vi "NyquistTrimCoefficients.vi"(7 "Cutoff type":string(combo), 9 "InterpolatedCoefficients":dbl[](array[numeric])=[1.0, 0.9893, 1.019, 1.0269, 1.0344, 1.0416, 1.0487, 1.0558, 1.0628, 1.0701, 1.0776, 1.0854, 1.0937, 1.1026, 1.1121, 1.1224, 1.1336, 1.1457, 1.1589, 1.1733, 1.189, 1.2061, 1.2246, 1.2447, 1.2662, 1.289, 1.3129, 1.3376, 1.3632, 1.3892, 1.4157, 1.4425, 1.4693, 1.496, 1.5226, 1.5491, 1.5754, 1.6016, 1.6277, 1.6535, 1.6792, 1.7046, 1.7298, 1.7548, 1.7794, 1.8033, 1.8263, 1.8483, 1.869, 1.8882, 1.9058, 1.9215, 1.935, 1.9464, 1.9556, 1.9628, 1.9684, 1.9723, 1.9748, 1.9762, 1.9765, 1.9759, 1.9748, 1.9731, 1.9711, 1.9689, 1.9667, 1.9646, 1.9628, 1.9614, 1.9606, 1.9605, 1.9612, 1.963, 1.9657, 1.9693, 1.9738, 1.979, 1.9848, 1.9913, 1.9983, 2.0059, 2.0138, 2.0221, 2.0308, 2.0401, 2.05, 2.0607, 2.0722, 2.0847, 2.0983, 2.113, 0.0, 0.0, 0.0, 0.0, 0.0, 0.0, 0.0, 0.0, 0.0, 0.0, 0.0, 0.0, 0.0, 0.0, 0.0, 0.0, 0.0, 0.0, 0.0, 0.0, 0.0, 0.0, 0.0, 0.0, 0.0, 0.0, 0.0, 0.0, 0.0, 0.0, 0.0, 0.0, 0.0, 0.0, 0.0, 0.0, 0.0, 0.0, 0.0, 0.0, 0.0, 0.0, 0.0, 0.0, 0.0, 0.0, 0.0, 0.0, 0.0, 0.0, 0.0, 0.0], 10 "Frequencies":dbl[](array[numeric])=[1.0, 0.9893, 1.019, 1.0269, 1.0344, 1.0416, 1.0487, 1.0558, 1.0628, 1.0701, 1.0776, 1.0854, 1.0937, 1.1026, 1.1121, 1.1224, 1.1336, 1.1457, 1.1589, 1.1733, 1.189, 1.2061, 1.2246, 1.2447, 1.2662, 1.289, 1.3129, 1.3376, 1.3632, 1.3892, 1.4157, 1.4425, 1.4693, 1.496, 1.5226, 1.5491, 1.5754, 1.6016, 1.6277, 1.6535, 1.6792, 1.7046, 1.7298, 1.7548, 1.7794, 1.8033, 1.8263, 1.8483, 1.869, 1.8882, 1.9058, 1.9215, 1.935, 1.9464, 1.9556, 1.9628, 1.9684, 1.9723, 1.9748, 1.9762, 1.9765, 1.9759, 1.9748, 1.9731, 1.9711, 1.9689, 1.9667, 1.9646, 1.9628, 1.9614, 1.9606, 1.9605, 1.9612, 1.963, 1.9657, 1.9693, 1.9738, 1.979, 1.9848, 1.9913, 1.9983, 2.0059, 2.0138, 2.0221, 2.0308, 2.0401, 2.05, 2.0607, 2.0722, 2.0847, 2.0983, 2.113, 0.0, 0.0, 0.0, 0.0, 0.0, 0.0, 0.0, 0.0, 0.0, 0.0, 0.0, 0.0, 0.0, 0.0, 0.0, 0.0, 0.0, 0.0, 0.0, 0.0, 0.0, 0.0, 0.0, 0.0, 0.0, 0.0, 0.0, 0.0, 0.0, 0.0, 0.0, 0.0, 0.0, 0.0, 0.0, 0.0, 0.0, 0.0, 0.0, 0.0, 0.0, 0.0, 0.0, 0.0, 0.0, 0.0, 0.0, 0.0, 0.0, 0.0, 0.0, 0.0], 11 "fs (Hz)":dbl) -> (1 "NyquistLimitedCoefficients":dbl[](array[numeric])=[1.0, 0.9893, 1.019, 1.0269, 1.0344, 1.0416, 1.0487, 1.0558, 1.0628, 1.0701, 1.0776, 1.0854, 1.0937, 1.1026, 1.1121, 1.1224, 1.1336, 1.1457, 1.1589, 1.1733, 1.189, 1.2061, 1.2246, 1.2447, 1.2662, 1.289, 1.3129, 1.3376, 1.3632, 1.3892, 1.4157, 1.4425, 1.4693, 1.496, 1.5226, 1.5491, 1.5754, 1.6016, 1.6277, 1.6535, 1.6792, 1.7046, 1.7298, 1.7548, 1.7794, 1.8033, 1.8263, 1.8483, 1.869, 1.8882, 1.9058, 1.9215, 1.935, 1.9464, 1.9556, 1.9628, 1.9684, 1.9723, 1.9748, 1.9762, 1.9765, 1.9759, 1.9748, 1.9731, 1.9711, 1.9689, 1.9667, 1.9646, 1.9628, 1.9614, 1.9606, 1.9605, 1.9612, 1.963, 1.9657, 1.9693, 1.9738, 1.979, 1.9848, 1.9913, 1.9983, 2.0059, 2.0138, 2.0221, 2.0308, 2.0401, 2.05, 2.0607, 2.0722, 2.0847, 2.0983, 2.113, 0.0, 0.0, 0.0, 0.0, 0.0, 0.0, 0.0, 0.0, 0.0, 0.0, 0.0, 0.0, 0.0, 0.0, 0.0, 0.0, 0.0, 0.0, 0.0, 0.0, 0.0, 0.0, 0.0, 0.0, 0.0, 0.0, 0.0, 0.0, 0.0, 0.0, 0.0, 0.0, 0.0, 0.0, 0.0, 0.0, 0.0, 0.0, 0.0, 0.0, 0.0, 0.0, 0.0, 0.0, 0.0, 0.0, 0.0, 0.0, 0.0, 0.0, 0.0, 0.0], 3 "NyquistFreq":dbl)   [LabVIEW 2011]
uses:
  <vilib>/Analysis/NI_AALBase.lvlib
panel:
  in  "cosineFadeLength":i32=12
  out "XY Graph":cluster{"Frequencies":dbl[], dbl[]}[](graph)
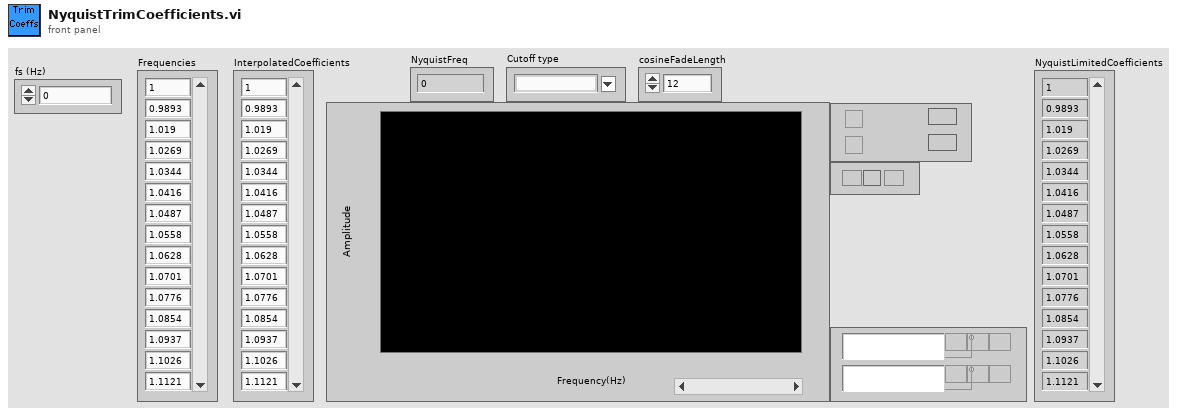
[diagram p1: front panel]
types:
  T1 = cluster{"Frequencies":dbl[], "InterpolatedCoefficients":dbl[]}
  T2 = cluster{"Frequencies":dbl[], "InterpolatedCoefficients":dbl[]}[]
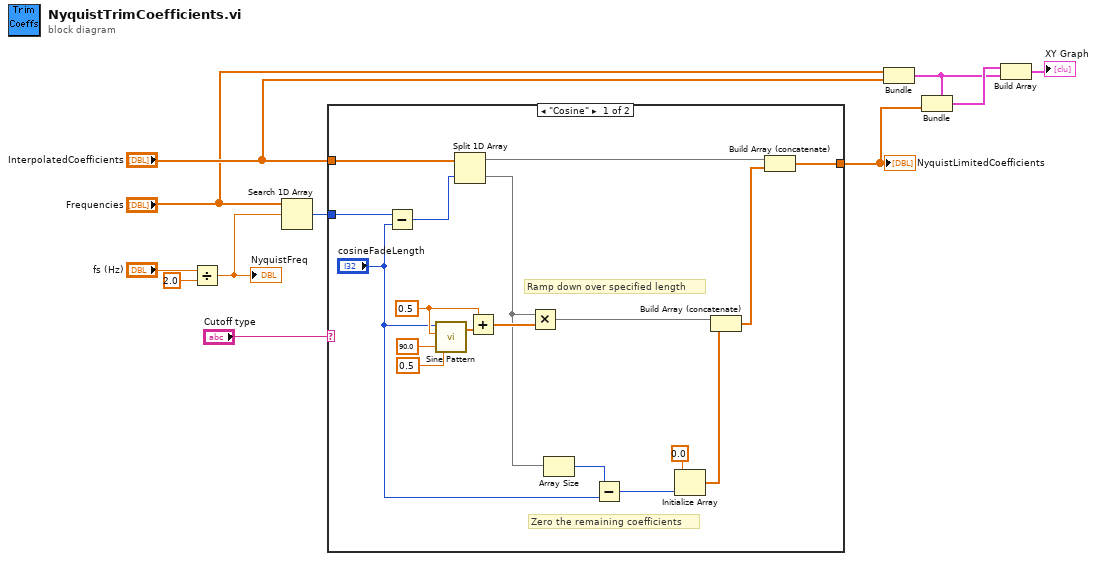
[diagram p0: block diagram]
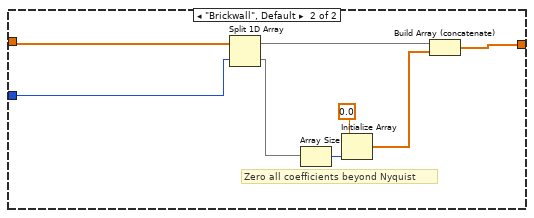
[diagram p2: hidden frame]
diagram:
  n1 = Divide(x="fs (Hz)", y=2.0) -> (x/y=w8:dbl)
  "NyquistFreq" <- w8
  n2 = Search 1D Array(1D array="Frequencies", element=w8) -> (index of element=w7:i32)  [unwired: 1 in]
  n3 = case shown="\"Cosine\"" "Cutoff type" {
    tunnel: "InterpolatedCoefficients" -> [w19 w35]
    tunnel: [w18 w31] -> w6
    tunnel: w7 -> [w17 w30]
    frame "Cosine" {
      w26 = 0.5 ("amplitude")
      # "Ramp down over specified length"
      # "Zero the remaining coefficients"
      n4 = Subtract(x=w17, y="cosineFadeLength") -> (x-y=w16:i32)
      n5 = call <vilib>:"Sine Pattern.vi"("cycles"=0.5, "phase(degrees)"=90.0, "amplitude"=w26, "samples"="cosineFadeLength") -> ("Sinusoidal Pattern"=w28:dbl[])  [unwired: 1 out]
      n6 = Split 1D Array(array=w19, index=w16) -> (first subarray=w20:dbl[], second subarray=w12:dbl[])
      n7 = Add(x=w26, y=w28) -> (x+y=w15:dbl[])
      n8 = Multiply(x=w12, y=w15) -> (x*y=w24:dbl[])
      n9 = Array Size(array=w12) -> (size(s)=w23:i32)
      n10 = Subtract(x=w23, y="cosineFadeLength") -> (x-y=w22:i32)
      n11 = Initialize Array(0.0 ("element"), w22) -> (w21:dbl[])
      n12 = Build Array (concatenate)(w24, w21) -> (w14:dbl[])
      n13 = Build Array (concatenate)(w20, w14) -> (w18:dbl[])
    }
    frame "Brickwall", Default {
      # "Zero all coefficients beyond Nyquist"
      n14 = Split 1D Array(array=w35, index=w30) -> (first subarray=w32:dbl[], second subarray=w34:dbl[])
      n15 = Array Size(array=w34) -> (size(s)=w37:i32)
      n16 = Initialize Array(0.0 ("element"), w37) -> (w33:dbl[])
      n17 = Build Array (concatenate)(w32, w33) -> (w31:dbl[])
    }
  }
  "NyquistLimitedCoefficients" <- w6
  n18 = Bundle("Frequencies"="Frequencies", "InterpolatedCoefficients"="InterpolatedCoefficients") -> (w1:T1)  [unwired: 1 in]
  n19 = Bundle(cluster=w1, "InterpolatedCoefficients"=w6) -> (w2:T1)  [unwired: 1 in]
  n20 = Build Array(w2, w1) -> (→"XY Graph":T2)
